vi "Get SMO LogTime.vi"(8 "error in (no error)":errorcluster, 11 "Instrument in":refnum<class "Instrument.lvclass">) -> (0 "error out":errorcluster, 2 "LogTime":T1=10000, 3 "Instrument out":refnum<class "Instrument.lvclass">)   [LabVIEW 2019, in "Instrument.lvclass"]
doc: "Override this VI to return the default logging period of your Instrument. This value can also be updated after your Instrument instance is created by calling \"Instrument.updateLogTime.vi\""
uses:
  Instrument.lvclass
  Typedefs/PrivateEvents--LogTime.ctl
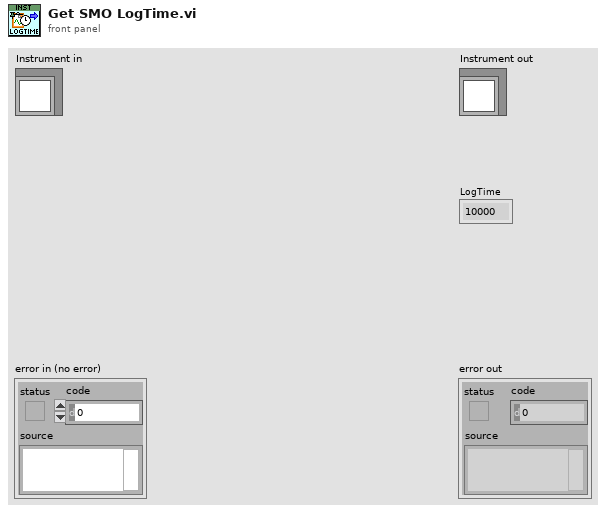
[diagram p1: front panel]
types:
  T1 = typedef "Instrument.lvclass/PrivateEvents--LogTime.ctl" = u32
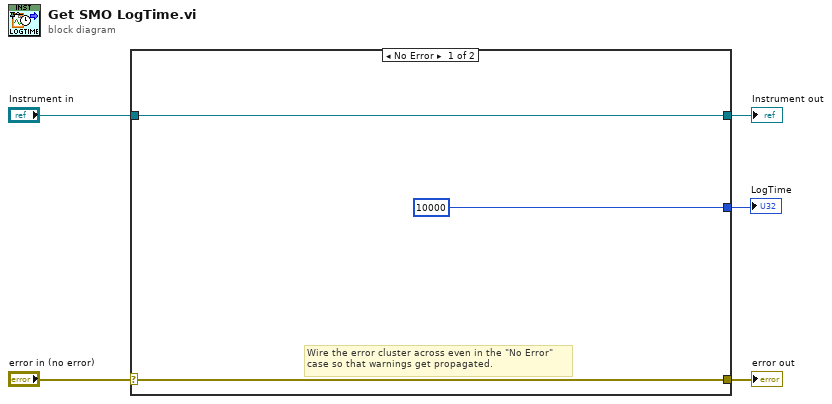
[diagram p0: block diagram]
diagram:
  n1 = case shown="No Error" "error in (no error)" {
    selector: "error in (no error)" -> [w8 w10]
    tunnel: [w8 w10] -> w4
    tunnel: [w7 w9] -> w2
    tunnel: "Instrument in" -> [w7 w9]
    tunnel: [T1 10000 ("LogTime") _] -> w1
    frame No Error {
      # "Wire the error cluster across even in the \"No Error\"\ncase so that warnings get propagated."
    }
    frame Error {
    }
  }
  "error out" <- w4
  "Instrument out" <- w2
  "LogTime" <- w1
